vi "Load INL PID Run Data.vi"(8 "error in":errorcluster, 10 "run number":i32, 11 "class objects":T1) -> (0 "error out":errorcluster, 3 "class objects":T1)   [LabVIEW 2011]
uses:
  Controls/Class Objects.ctl
  Modules/File/Configuration/Configuration.lvclass
  Modules/Hardware/Power Supply/Power Supply.lvclass
  Modules/Hardware/Mass Flow Controller/Mass Flow Controller.lvclass
  Modules/Hardware/PID/PID.lvclass
  Modules/Hardware/Valve Controller/Valve Controller.lvclass
  Modules/Hardware/Multimeter/Multimeter.lvclass
  Modules/Hardware/Vapour Generator/Vapour Generator.lvclass
  Modules/File/TDMS/TDMS.lvclass
  Modules/File/TDMS/Parameter Data Type.ctl
  Modules/File/TDMS/File Level.ctl
  Functional Global Data/Run Data.ctl
  Controls/TDMS File Handling.ctl
  Controls/User Interface Action.ctl
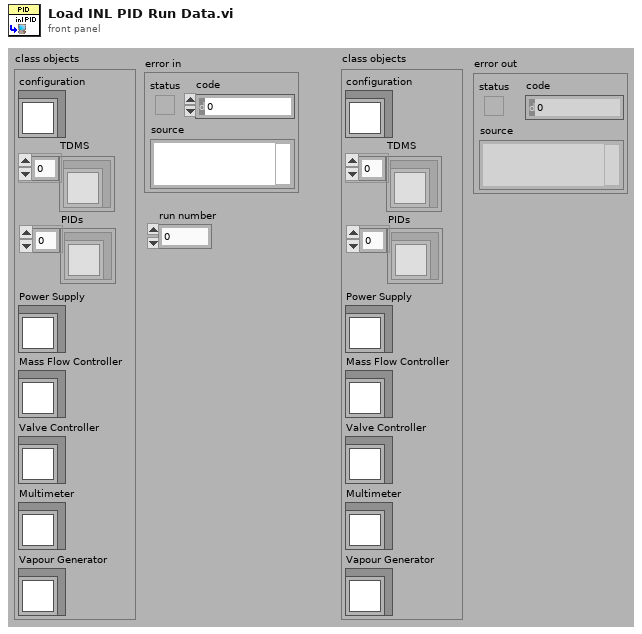
[diagram p1: front panel]
types:
  T1 = typedef "Class Objects.ctl" = cluster{"configuration":refnum<class "Configuration.lvclass">, "TDMS":refnum<class "TDMS.lvclass">[], "Power Supply":refnum<class "Power Supply.lvclass">, "Mass Flow Controller":refnum<class "Mass Flow Controller.lvclass">, "Valve Controller":refnum<class "Valve Controller.lvclass">, "Multimeter":refnum<class "Multimeter.lvclass">, "Vapour Generator":refnum<class "Vapour Generator.lvclass">, "PIDs":refnum<class "PID.lvclass">[]}
  T2 = typedef "TDMS.lvclass/Parameter Data Type.ctl" = enum16{"Boolean", "U32", "I32", "Double", "String", "Path"}
  T3 = typedef "TDMS.lvclass/File Level.ctl" = enum16{"File", "Group", "Channel"}
  T4 = typedef "Run Data.ctl" = enum16{"Initialize", "Add Sample Channel", "Set Run", "Get Number of Runs", "Set Run Params", "Get Spectrum", "Get Run Params", "Get Sample Params", "Get History", "Get Averaged History", "Get Run Param Names", "Set Run Param Names", "Get Sample Param Names", "Set Sample Param Names", "Get MFC Flow Rate Challenge Profile", "Get History Average"}
  T5 = typedef "TDMS File Handling.ctl" = enum16{"Add TDMS File", "Get Active TDMS File", "Set Active TDMS File", "Set Active TDMS File Index"}
  T6 = typedef "User Interface Action.ctl" = enum16{"Initialize", "Data Acquisition Disable", "Data View Disable", "Sample Set", "Sample Set 2D Data", "Sample Set x0 & dx", "Sample Add", "Sample Set Cursor", "Sample Set Offset & Multiplier", "Sample Set Axis Labels", "Sample Parameters Disabled", "Sample Parameters Update", "Run Update", "Run Set Offset & Multiplier", "Run Set Axis Labels", "Run Set Cursor", "Run Set Disabled", "Run Parameters Update", "Run Parameters Disabled", "Run Number Set", "Run Number Set Range", "Run Number Set Disabled", "Sample Number Set", "Sample Number Set Range", "Notes Set Value", "Update Plot", "Set Plot Parameters", "Update Concentration Plot", "Time Set", "Clear DAQ Display", "Clear Analysis Display", "Status Bar Set", "Progress Bar Set", "Display Mode Set", "Experiment Type Set", "Analysis Plot Average Set", "Stop"}
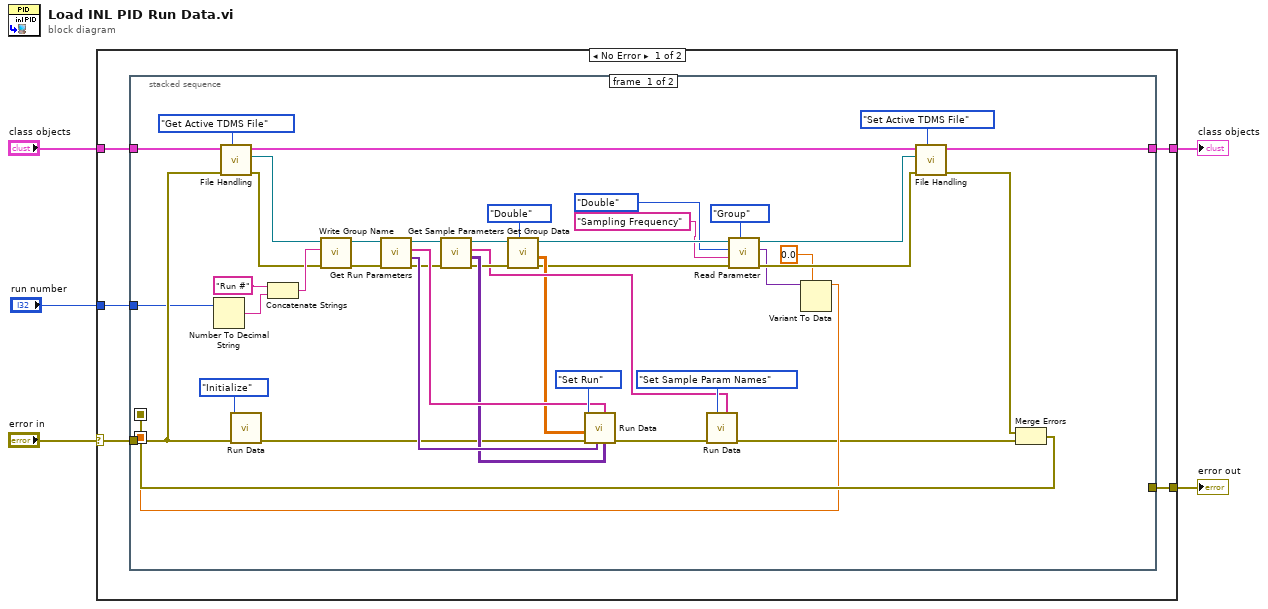
[diagram p0: block diagram]
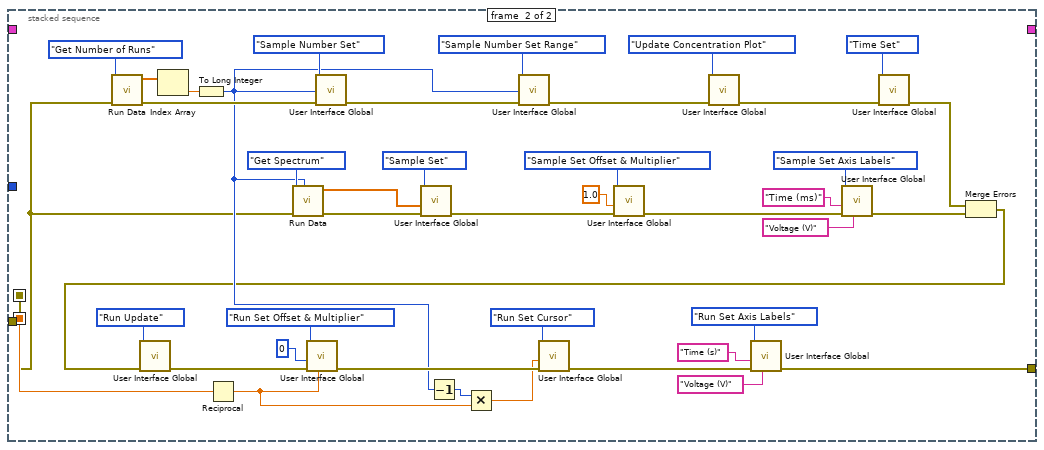
[diagram p2: hidden frame]
diagram:
  n1 = case shown="No Error" "error in" {
    selector: "error in" -> [w8 w95]
    tunnel: "class objects" -> [w10 w96]
    tunnel: "run number" -> [w7 _]
    tunnel: [w6 w95] -> w3
    tunnel: [w9 w96] -> w2
    frame No Error {
      n2 = stacked-sequence {
        seq-local: [w22 _] -> [_ w56]
        seq-local: [w12 _] -> [_ w80]
        tunnel: w10 -> [w50 _]
        tunnel: [w46 _] -> w9
        tunnel: w8 -> [w42 _]
        tunnel: w7 -> [w32 _]
        tunnel: [_ w59] -> w6
        frame #0 {
          n3 = Number To Decimal String(number=w32) -> (decimal integer string=w33:string)  [unwired: 1 in]
          n4 = call "File Handling.vi"("TDMS File Handling"=TDMS_File_Handling."Get Active TDMS File", "error in"=w42, "Class objects"=w50) -> ("error out"=w30:errorcluster, "TDMS File"=w49:refnum<class "TDMS.lvclass">, "Class objects"=w48:T1)  [unwired: 6 in]
          n5 = call "Run Data.vi"("error in"=w42, "action"=Run_Data."Initialize" ("Action")) -> ("error out"=w25:errorcluster)  [unwired: 6 in, 3 out]
          n6 = Concatenate Strings("Run #" ("string"), w33) -> (w31:string)
          n7 = call-dynamic "Write Group Name.vi"("error in (no error)"=w30, "Group Name"=w31, "TDMS in"=w49) -> ("error out"=w26:errorcluster, "TDMS out"=w24:refnum<class "TDMS.lvclass">)  [unwired: 7 in]
          n8 = call-dynamic "Get Run Parameters.vi"("error in"=w26, "TDMS in"=w24) -> ("error out"=w39:errorcluster, "run params"=w41:variant[], "param names"=w40:string[], "TDMS out"=w38:refnum<class "TDMS.lvclass">)  [unwired: 6 in]
          n9 = call-dynamic "Get Sample Parameters.vi"("error in"=w39, "TDMS in"=w38) -> ("error out"=w35:errorcluster, "sample params"=w36:variant[][], "sample param names"=w27:string[], "TDMS out"=w37:refnum<class "TDMS.lvclass">)  [unwired: 6 in]
          n10 = call "Get Group Data.vi"("data type"=enum16{"I16", "Double"}."Double" ("Data Type"), "error in"=w35, "TDMS in"=w37) -> ("error out"=w19:errorcluster, "double group data"=w23:dbl[][], "TDMS out"=w21:refnum<class "TDMS.lvclass">)  [unwired: 3 in, 3 out]
          n11 = call "Run Data.vi"("Params 2D IN"=w36, "Param Names IN"=w40, "Params 1D IN"=w41, "error in"=w25, "Data 2D IN"=w23, "action"=Run_Data."Set Run" ("Action")) -> ("error out"=w28:errorcluster)  [unwired: 2 in, 3 out]
          n12 = call "Run Data.vi"("Param Names IN"=w27, "error in"=w28, "action"=Run_Data."Set Sample Param Names") -> ("error out"=w11:errorcluster)  [unwired: 5 in, 3 out]
          n13 = call-dynamic "Read Parameter.vi"("file level"=File_Level."Group", "error in"=w19, "Parameter Name"="Sampling Frequency", "data type"=Parameter_Data_Type."Double", "TDMS in"=w21) -> ("error out"=w16:errorcluster, "parameter"=w14:variant, "TDMS out"=w15:refnum<class "TDMS.lvclass">)  [unwired: 3 in, 1 out]
          n14 = Variant To Data(type=0.0, Variant=w14) -> (data=w12:dbl)  [unwired: 1 in, 1 out]
          n15 = call "File Handling.vi"("TDMS File Handling"=TDMS_File_Handling."Set Active TDMS File", "error in"=w16, "TDMS File"=w15, "Class objects"=w48) -> ("error out"=w47:errorcluster, "Class objects"=w46:T1)  [unwired: 5 in, 1 out]
          n16 = Merge Errors(w47, w11) -> (w22:errorcluster)
        }
        frame #1 {
          n17 = call "Run Data.vi"("error in"=w56, "action"=Run_Data."Get Number of Runs" ("Action")) -> ("error out"=w65:errorcluster, "Data 1D OUT"=w64:dbl[])  [unwired: 6 in, 2 out]
          n18 = Index Array(array=w64) -> (element=w63:dbl)  [unwired: 1 in]
          n19 = To Long Integer(number=w63) -> (32bit integer=w61:i32)
          n20 = Reciprocal(x=w80) -> (1/x=w78:dbl)
          n21 = call "Run Data.vi"("Index Number"=w61, "error in"=w56, "action"=Run_Data."Get Spectrum" ("Action")) -> ("error out"=w94:errorcluster, "Data 1D OUT"=w91:dbl[])  [unwired: 5 in, 2 out]
          n22 = call "User Interface Global.vi"("error in"=w65, "data1"=w61, "action"=User_Interface_Action."Sample Number Set" ("Action")) -> ("error out"=w82:errorcluster)  [unwired: 8 in]
          n23 = call "User Interface Global.vi"("error in"=w94, "data1"=w91, "action"=User_Interface_Action."Sample Set" ("Action")) -> ("error out"=w89:errorcluster)  [unwired: 8 in]
          n24 = Decrement(x=w61) -> (x-1=w76:i32)
          n25 = Multiply(x=w76, y=w78) -> (x*y=w77:dbl)
          n26 = call "User Interface Global.vi"("error in"=w82, "data1"=w61, "action"=User_Interface_Action."Sample Number Set Range" ("Action")) -> ("error out"=w54:errorcluster)  [unwired: 8 in]
          n27 = call "User Interface Global.vi"("error in"=w89, "data1"=1.0, "action"=User_Interface_Action."Sample Set Offset & Multiplier" ("Action")) -> ("error out"=w69:errorcluster)  [unwired: 8 in]
          n28 = call "User Interface Global.vi"("error in"=w54, "action"=User_Interface_Action."Update Concentration Plot" ("Action")) -> ("error out"=w55:errorcluster)  [unwired: 9 in]
          n29 = call "User Interface Global.vi"("data2"="Voltage (V)", "error in"=w69, "data1"="Time (ms)", "action"=User_Interface_Action."Sample Set Axis Labels" ("Action")) -> ("error out"=w62:errorcluster)  [unwired: 7 in]
          n30 = call "User Interface Global.vi"("error in"=w55, "action"=User_Interface_Action."Time Set") -> ("error out"=w53:errorcluster)  [unwired: 9 in]
          n31 = Merge Errors(w53, w62) -> (w60:errorcluster)
          n32 = call "User Interface Global.vi"("error in"=w60, "action"=User_Interface_Action."Run Update" ("Action")) -> ("error out"=w81:errorcluster)  [unwired: 9 in]
          n33 = call "User Interface Global.vi"("data2"=w78, "error in"=w81, "data1"=0, "action"=User_Interface_Action."Run Set Offset & Multiplier" ("Action")) -> ("error out"=w83:errorcluster)  [unwired: 7 in]
          n34 = call "User Interface Global.vi"("error in"=w83, "data1"=w77, "action"=User_Interface_Action."Run Set Cursor" ("Action")) -> ("error out"=w74:errorcluster)  [unwired: 8 in]
          n35 = call "User Interface Global.vi"("data2"="Voltage (V)", "error in"=w74, "data1"="Time (s)", "action"=User_Interface_Action."Run Set Axis Labels" ("Action")) -> ("error out"=w59:errorcluster)  [unwired: 7 in]
        }
      }
    }
    frame Error {
    }
  }
  "class objects" <- w2
  "error out" <- w3
